vi "Gen NextState (SubVI).vi"(10 "Action":i32, 11 "State":i32) -> (3 "Next State":i32)   [LabVIEW 2013]
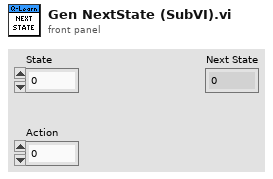
[diagram p1: front panel]
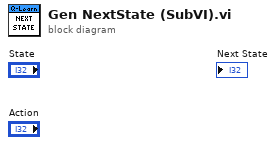
[diagram p0: block diagram]
diagram:
